vi "front-time(SubVI).vi"(11 "x":i32) -> ()   [LabVIEW 2016]
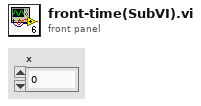
[diagram p1: front panel]
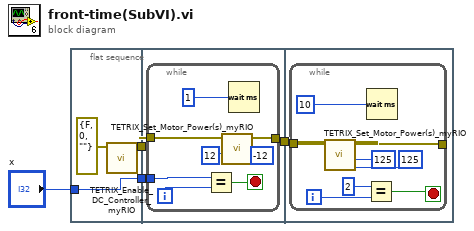
[diagram p0: block diagram]
diagram:
  n1 = flat-sequence {
    tunnel: [w6] -> w4
    tunnel: [w5] -> w3
    tunnel: "x" -> [w5]
    tunnel: w4 -> [w10]
    tunnel: [w9] -> w2
    tunnel: w3 -> [w8]
    tunnel: w2 -> [w19]
    frame #0 {
      n2 = call <vilib>:"TETRIX_Enable_DC_Controller_myRIO.vi"("Error/Flow In"=errorcluster {"status"=FALSE, "code"=0, "source"=""}) -> ("Error/Flow Out"=w6:errorcluster)  [unwired: 6 in]
    }
    frame #1 {
      n3 = while {
        tunnel: w10 -> [w17]
        tunnel: [w16] -> w9
        tunnel: w8 -> [w11]
        i -> [w15]
        stop <- w12 stop-if-true
        n4 = Equal?(x=w11, y=w15) -> (x = y?=w12:bool)
        n5 = call <vilib>:"TETRIX_Set_Motor_Power(s)_myRIO.vi"("Motor 2 Power (-100 to 100)  0 = Coast Stop  125 = Brake Stop"=i8 -12, "Motor 1 Power (-100 to 100)  0 = Coast Stop  125 = Brake Stop"=i8 12, "Error/Flow In"=w17) -> ("Error/Flow Out"=w16:errorcluster)  [unwired: 4 in]
        n6 = Wait (ms)(milliseconds to wait=u32 1) -> ()  [unwired: 1 out]
      }
    }
    frame #2 {
      n7 = while {
        tunnel: w19 -> [w23]
        tunnel: [w22] -> _
        i -> [w26]
        stop <- w21 stop-if-true
        n8 = call <vilib>:"TETRIX_Set_Motor_Power(s)_myRIO.vi"("Motor 2 Power (-100 to 100)  0 = Coast Stop  125 = Brake Stop"=i8 125, "Motor 1 Power (-100 to 100)  0 = Coast Stop  125 = Brake Stop"=i8 125, "Error/Flow In"=w23) -> ("Error/Flow Out"=w22:errorcluster)  [unwired: 4 in]
        n9 = Equal?(x=2, y=w26) -> (x = y?=w21:bool)
        n10 = Wait (ms)(milliseconds to wait=u32 10) -> ()  [unwired: 1 out]
      }
    }
  }
